vi "GPS to XY Conversion.vi"(2 "Reference Latitude":dbl, 3 "Reference Longitude":dbl, 4 "Current Latitude":dbl, 5 "Current Longitude":dbl) -> (0 "y":dbl, 1 "x":dbl)   [LabVIEW 2009]
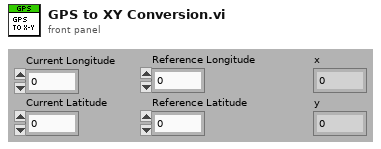
[diagram p1: front panel]
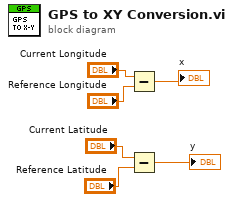
[diagram p0: block diagram]
diagram:
  n1 = Subtract(x="Current Longitude", y="Reference Longitude") -> (x-y=→"x":dbl)
  n2 = Subtract(x="Current Latitude", y="Reference Latitude") -> (x-y=→"y":dbl)
